vi "GetFeatures.vi"(6 "supported metrics":string[](array[string]), 7 "high rate":bool, 8 "error in (no error)":errorcluster, 9 "Metric Cache":variant, 11 "ChannelModel":T5) -> (0 "error out":errorcluster, 2 "Chanel":T1)   [LabVIEW 2017, in "AnalysisHelper.lvlib"]
uses:
  <vilib>/addons/InsightCM/Utilities/Analysis/Shared/AnalysisHelper.lvlib
  <vilib>/addons/InsightCM/MessageBus/Base/controls/R2_Channel.ctl
  <vilib>/addons/InsightCM/MessageBus/Base/controls/KeyValuePair.ctl
  <vilib>/addons/InsightCM/MessageBus/Base/controls/Metric.ctl
  <vilib>/addons/InsightCM/Utilities/Analysis/Shared/controls/Channel.ctl
  <vilib>/addons/InsightCM/Utilities/Analysis/Shared/controls/SpeedType.ctl
  <vilib>/addons/InsightCM/Utilities/Analysis/Shared/controls/Feature.ctl
  <vilib>/addons/InsightCM/Utilities/Analysis/Shared/controls/AmplitudeScale.ctl
  <vilib>/addons/InsightCM/Utilities/Tdms/Tdms.lvlib
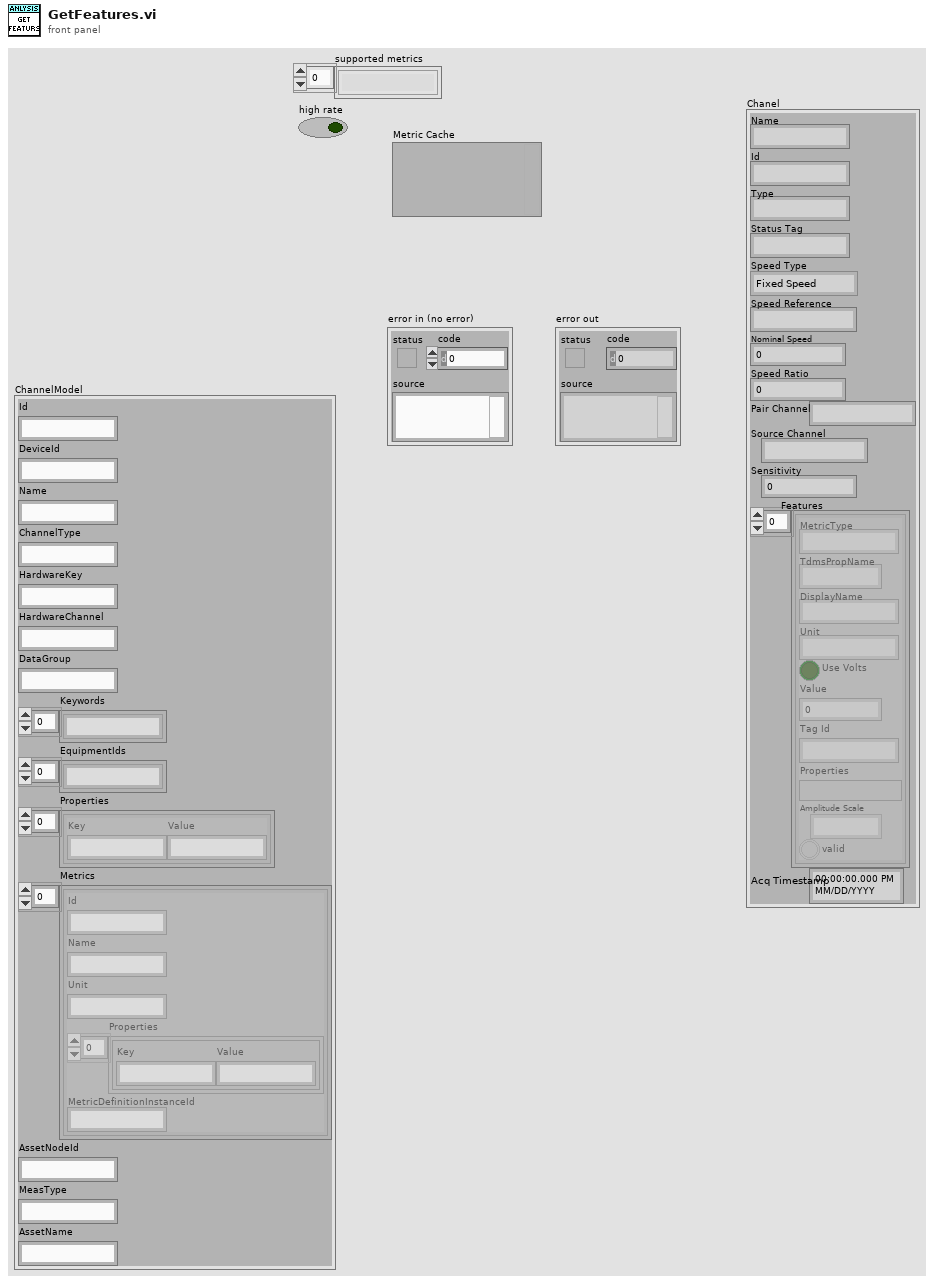
[diagram p1: front panel]
types:
  T1 = typedef "AnalysisHelper.lvlib/Channel.ctl" = cluster{"Name":string, "Id":string, "Type":string, "Status Tag":string, "Speed Type":T2, "Speed Reference":string, "Nominal Speed":dbl, "Speed Ratio":dbl, "Pair Channel":string, "Source Channel":string, "Sensitivity":dbl, "Features":T3[], "Acq Timestamp":timestamp}
  T2 = typedef "AnalysisHelper.lvlib/SpeedType.ctl" = enum16{"Fixed Speed", "Tachometer", "From Map"}
  T3 = typedef "AnalysisHelper.lvlib/Feature.ctl" = cluster{"MetricType":string, "TdmsPropName":string, "DisplayName":string, "Unit":string, "Use Volts":bool, "Value":dbl, "Tag Id":string, "Properties":variant, "Amplitude Scale":T4, "valid":bool}
  T4 = typedef "AnalysisHelper.lvlib/AmplitudeScale.ctl" = enum16{"rms", "peak", "pk-pk"}
  T5 = typedef "R2_Channel.ctl" = cluster{"Id":string, "DeviceId":string, "Name":string, "ChannelType":string, "HardwareKey":string, "HardwareChannel":string, "DataGroup":string, "Keywords":string[], "EquipmentIds":string[], "Properties":T6[], "Metrics":T7[], "AssetNodeId":string, "MeasType":string, "AssetName":string}
  T6 = typedef "KeyValuePair.ctl" = cluster{"Key":string, "Value":string}
  T7 = typedef "Metric.ctl" = cluster{"Id":string, "Name":string, "Unit":string, "Properties":T6[], "MetricDefinitionInstanceId":string}
  T8 = typedef "AnalysisHelper.lvlib/BandConfig.ctl" = cluster{"High":dbl, "Low":dbl, "Domain":T9, "Calculation":T10}
  T9 = typedef "AnalysisHelper.lvlib/BandDomain.ctl" = enum16{"Frequency", "CPM", "Orders"}
  T10 = typedef "AnalysisHelper.lvlib/BandCalculation.ctl" = enum16{"Total", "Max", "Phase"}
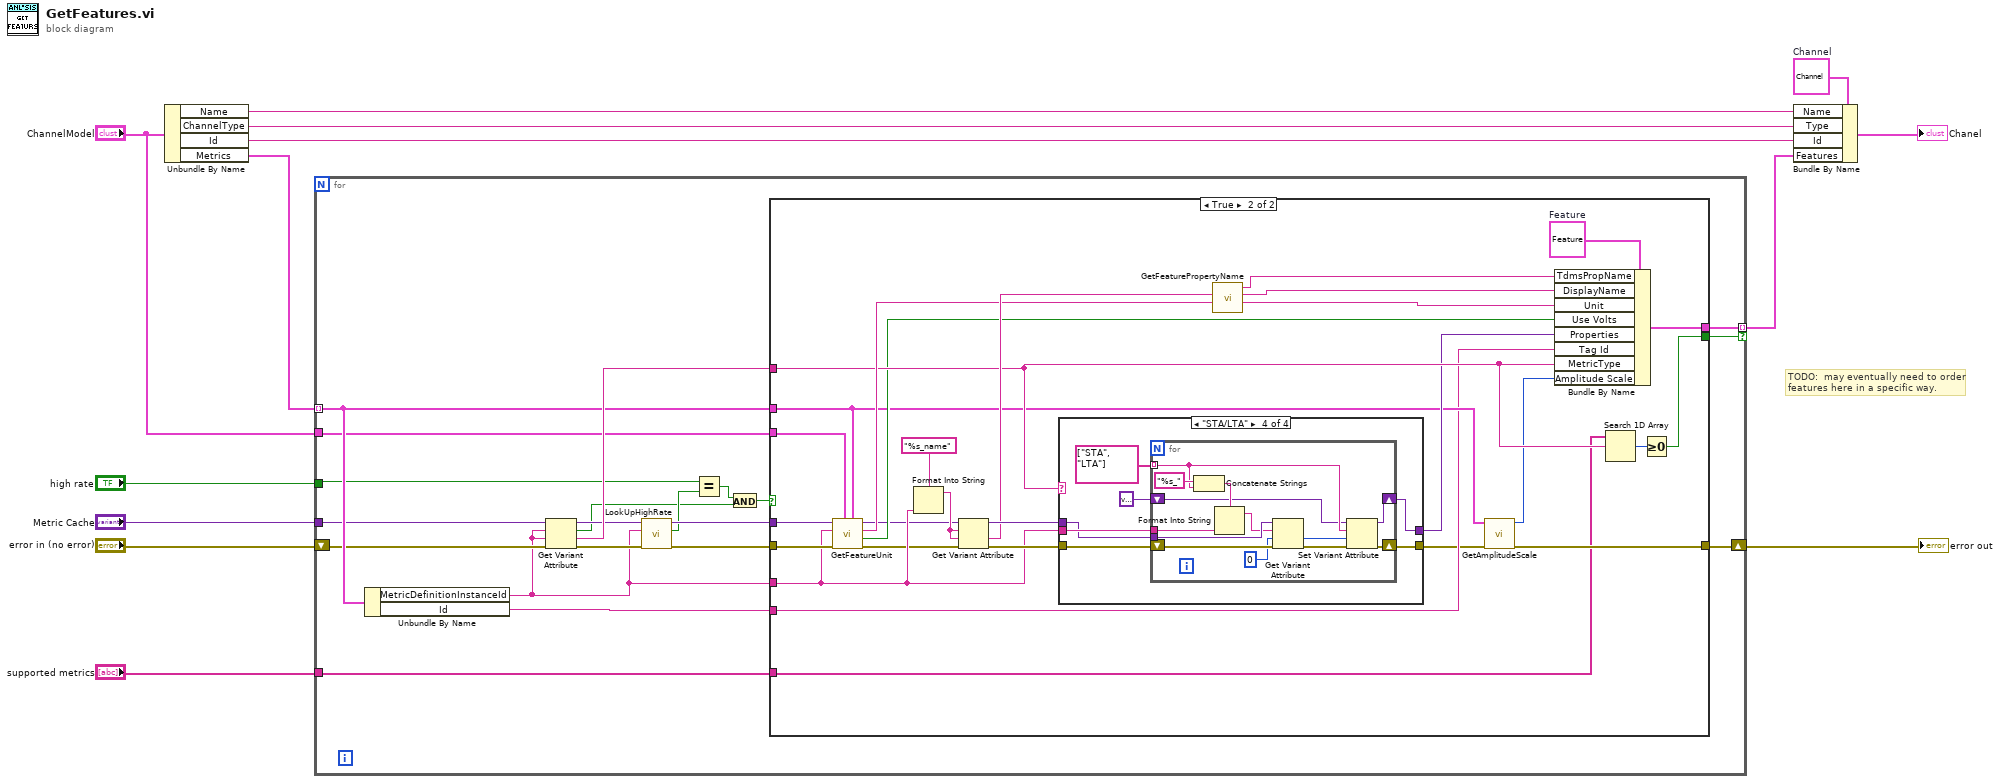
[diagram p0: block diagram]
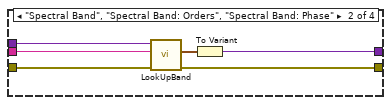
[diagram p4: hidden frame]
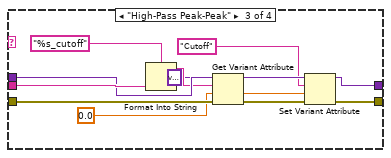
[diagram p5: hidden frame]
diagram:
  w11 = T1 {"Name"="", "Id"="", "Type"="", "Status Tag"="", "Speed Type"=enum."Fixed Speed", "Speed Reference"="", "Nominal Speed"=0.0, "Speed Ratio"=0.0, "Pair Channel"="", "Source Channel"="", "Sensitivity"=0.0, "Features"=[], "Acq Timestamp"=timestamp(0 s since 1904-01-01)}  # Channel
  # "TODO:  may eventually need to order\nfeatures here in a specific way."
  n1 = Unbundle By Name("ChannelModel") -> ("Name"=w10:string, "ChannelType"=w6:string, "Id"=w7:string, "Metrics"=w9:T7[])
  n2 = for {
    tunnel: "Metric Cache" -> [w26]
    tunnel: w9 -> [w29] mode=indexing
    tunnel: [w31] -> w8 mode=indexing if=w30
    shift-right: [w32] -> w4
    shift-left: "error in (no error)" -> [w27]
    tunnel: "ChannelModel" -> [w25]
    tunnel: "supported metrics" -> [w24]
    tunnel: "high rate" -> [w18]
    n3 = Unbundle By Name(w29) -> ("MetricDefinitionInstanceId"=w19:string, "Id"=w28:string)
    n4 = Get Variant Attribute(Variant=w26, name=w19, default value (empty Variant)=w19, error in=w27) -> (duplicate Variant=w23:variant, found=w14:bool, value=w33:string, error out=w21:errorcluster)
    n5 = call <vilib>:"LookUpHighRate.vi"("error in (no error)"=w21, "MetricDefinitionInstanceId"=w19, "Metric Cache"=w23) -> ("error out"=w20:errorcluster, "high rate"=w17:bool, "Metric Cache Out"=w22:variant)  [unwired: 6 in]
    n6 = Equal?(x=w18, y=w17) -> (x = y?=w15:bool)
    n7 = And(x=w15, y=w14) -> (x .and. y?=w16:bool)
    n8 = case shown="True" w16 {
      tunnel: w20 -> [w34 w52]
      tunnel: w33 -> [_ w49]
      tunnel: w28 -> [_ w36]
      tunnel: w22 -> [_ w51]
      tunnel: [w34 w40] -> w32
      tunnel: [_ w59] -> w31
      tunnel: [_ w47] -> w30
      tunnel: w19 -> [_ w46]
      tunnel: w29 -> [_ w39]
      tunnel: w25 -> [_ w45]
      tunnel: w24 -> [_ w37]
      frame False {
        # "Metric does not match the \"rate\", meaning this\nis a high rate feature, but we're in the low rate\nconfig (or vise versa).\nOR\nMetric Def Instance Id not found in cache"
      }
      frame True {
        w62 = T3 {"MetricType"="", "TdmsPropName"="", "DisplayName"="", "Unit"="", "Use Volts"=FALSE, "Value"=0.0, "Tag Id"="", "Properties"=variant(string ""), "Amplitude Scale"=enum."rms", "valid"=FALSE}  # Feature
        n9 = call <vilib>:"GetFeatureUnit.vi"("metric"=w39, "channel"=w45, "error in (no error)"=w52, "metric definitionInstance id"=w46, "metric cache in"=w51) -> ("error out"=w41:errorcluster, "use volts"=w43:bool, "unit"=w50:string, "metric cache out"=w42:variant)  [unwired: 3 in]
        n10 = Format Into String(format string="%s_name", w46) -> (resulting string=w60:string)  [unwired: 2 in, 1 out]
        n11 = Get Variant Attribute(Variant=w42, name=w60, default value (empty Variant)=w60, error in=w41) -> (duplicate Variant=w58:variant, value=w54:string, error out=w57:errorcluster)  [unwired: 1 out]
        n12 = case shown="\"STA/LTA\"" w49 {
          tunnel: w58 -> [_ w69 w79 w87]
          tunnel: w57 -> [w63 w68 w78 w86]
          tunnel: [_ w64 w75 w85] -> w44
          tunnel: w46 -> [_ w65 w80 w88]
          tunnel: [w63 w66 w74 w84] -> w35
          frame Default {
          }
          frame "Spectral Band", "Spectral Band: Orders", "Spectral Band: Phase" {
            n13 = call <vilib>:"LookUpBand.vi"("error in (no error)"=w68, "MetricDefinitionInstanceId"=w65, "Metric Cache"=w69) -> ("error out"=w66:errorcluster, "SpectralBand"=w67:T8)  [unwired: 6 in, 1 out]
            n14 = To Variant(anything=w67) -> (Variant=w64:variant)
          }
          frame "High-Pass Peak-Peak" {
            n15 = Format Into String(format string="%s_cutoff", w80) -> (resulting string=w77:string)  [unwired: 2 in, 1 out]
            n16 = Get Variant Attribute(Variant=w79, name=w77, default value (empty Variant)=sgl 0.0 ("default (0 DBL)"), error in=w78) -> (value=w72:sgl, error out=w73:errorcluster)  [unwired: 2 out]
            n17 = Set Variant Attribute(Variant=variant ("variant"), name="Cutoff", value=w72, error in=w73) -> (Variant out=w75:variant, error out=w74:errorcluster)  [unwired: 1 out]
          }
          frame "STA/LTA" {
            n18 = for {
              tunnel: w88 -> [w101]
              tunnel: w87 -> [w100]
              shift-right: [w95] -> w84
              shift-left: w86 -> [w99]
              tunnel: string[] ["STA", "LTA"] -> [w90] mode=indexing
              shift-right: [w96] -> w85
              shift-left: variant ("variant") -> [w89]
              n19 = Concatenate Strings("%s_" ("format string"), w90) -> (w91:string)
              n20 = Format Into String(format string=w91, w101) -> (resulting string=w98:string)  [unwired: 2 in, 1 out]
              n21 = Get Variant Attribute(Variant=w100, name=w98, default value (empty Variant)=0 ("default (0 DBL)"), error in=w99) -> (value=w93:i32, error out=w94:errorcluster)  [unwired: 2 out]
              n22 = Set Variant Attribute(Variant=w89, name=w90, value=w93, error in=w94) -> (Variant out=w96:variant, error out=w95:errorcluster)  [unwired: 1 out]
            }
          }
        }
        n23 = call <vilib>:"GetFeaturePropertyName.vi"("unit"=w50, "metric name"=w54) -> ("tdms unit value"=w55:string, "display name"=w56:string, "tdms property name"=w53:string)  [unwired: 7 in]
        n24 = call <vilib>:"GetAmplitudeScale.vi"("error in (no error)"=w35, "metric"=w39) -> ("error out"=w40:errorcluster, "amplitude scale"=w38:T4)  [unwired: 8 in]
        n25 = Bundle By Name(cluster=w62, "TdmsPropName"=w53, "DisplayName"=w56, "Unit"=w55, "Use Volts"=w43, "Properties"=w44, "Tag Id"=w36, "MetricType"=w49, "Amplitude Scale"=w38) -> (w59:T3)
        n26 = Search 1D Array(1D array=w37, element=w49) -> (index of element=w48:i32)  [unwired: 1 in]
        n27 = Greater Or Equal To 0?(x=w48) -> (x >= 0?=w47:bool)
      }
    }
  }
  "error out" <- w4
  n28 = Bundle By Name(cluster=w11, "Name"=w10, "Type"=w6, "Id"=w7, "Features"=w8) -> (→"Chanel":T1)
